vi "_Release JKISMQ.vi"(8 "Error in":errorcluster caption="Error in (no error)", 11 "JKISMQ":T1) -> (0 "Error out":errorcluster)   [LabVIEW 2014, in "JKI State Machine++.lvlib"]
uses:
  JKI State Machine++.lvlib
  _JKISMQ.ctl
  Typedef/_Cross JKISM State Data.ctl
  Typedef/_JKISM_MSG_TYPE.ctl
  Typedef/_Cross JKISM State Response.ctl
  Typedef/_JKISM_MODE.ctl
  _JKISMQFGVOPER.ctl
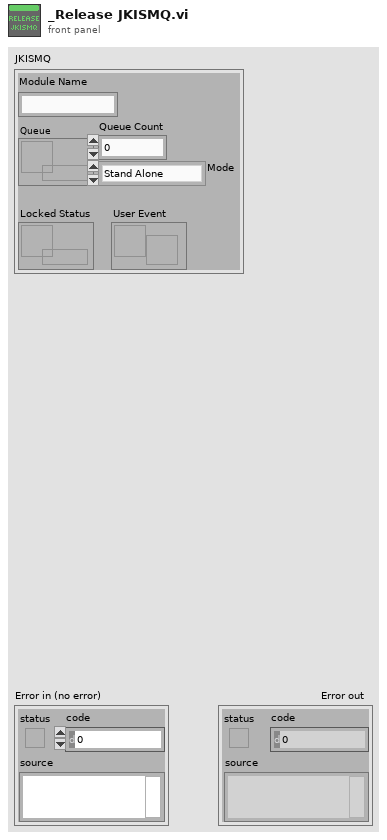
[diagram p1: front panel]
types:
  T1 = typedef "JKI State Machine++.lvlib/_JKISMQ.ctl" = cluster{"Module Name":string, "Queue":refnum<queue>, "Locked Status":refnum<data-value>, "Mode":T2, "User Event":refnum<user-event>, "Queue Count":i32}
  T2 = typedef "JKI State Machine++.lvlib/_JKISM_MODE.ctl" = enum16{"Stand Alone", "JKISM", "Action Worker"}
  T3 = typedef "JKI State Machine++.lvlib/_JKISMQFGVOPER.ctl" = enum16{"Get By Name", "List", "Check If Name Exists", "Release", "Module Status"}
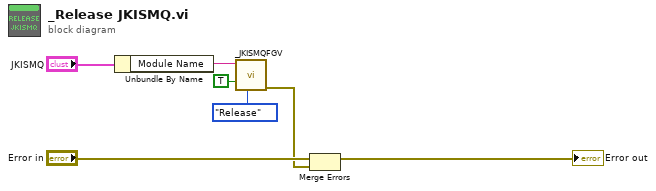
[diagram p0: block diagram]
diagram:
  n1 = Unbundle By Name("JKISMQ") -> ("Module Name"=w5:string)
  n2 = call "_JKISMQFGV.vi"(6:_JKISMQFGVOPER."Release", "create if not found? (T)"=TRUE, "Name(\"\" to use uuid) in"=w5) -> ("Error out"=w2:errorcluster)  [unwired: 5 in, 3 out]
  n3 = Merge Errors("Error in", w2) -> (→"Error out":errorcluster)
